vi "output.vi"(8 "error in (no error)":errorcluster, 10 "Output [on/off]":bool, 11 "PSP-603 in":refnum<class "PSP-603.lvclass">) -> (0 "error out":errorcluster, 3 "PSP-603 out":refnum<class "PSP-603.lvclass">)   [LabVIEW 2025, in "Power Supply.lvlib" / "PSP-603.lvclass"]
uses:
  PSP-603.lvclass
  PSP-603.lvclass/PSP-603.ctl
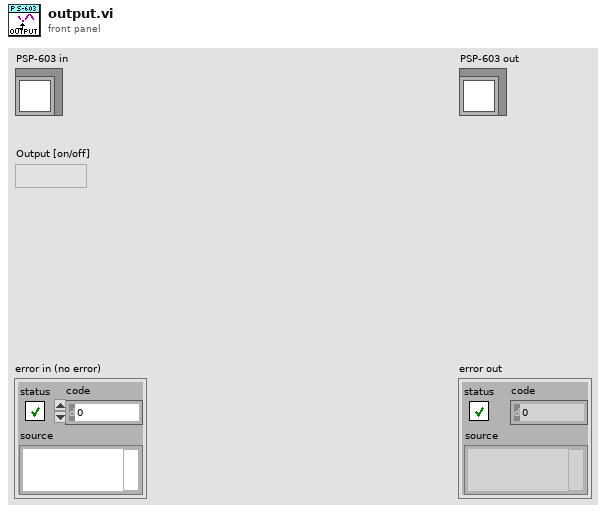
[diagram p1: front panel]
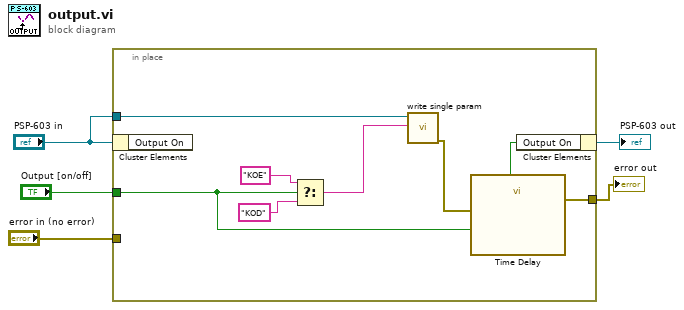
[diagram p0: block diagram]
diagram:
  n1 = in-place {
    in-place-border: "Output [on/off]" -> [w11]
    in-place-border: "PSP-603 in" -> [w12]
    in-place-border: "error in (no error)" -> [_]
    in-place-border: [w6] -> w1
    n2 = in-place-cluster #1("PSP-603 in") -> ()  [unwired: 1 out]
    n3 = Select(t="KOE" ("string"), s=w11, f="KOD" ("string")) -> (s? t:f=w8:string)
    n4 = call-dynamic "write single param.vi"("string"=w8, "PSP-603 in"=w12) -> ("error out"=w7:errorcluster)  [unwired: 8 in, 1 out]
    n5 = call "Time Delay"("error in (no error)"=w7) -> ("error out"=w6:errorcluster)  [unwired: 10 in]
    n6 = in-place-cluster #1("Output On"=w11) -> (→"PSP-603 out":refnum<class "PSP-603.lvclass">)
  }
  "error out" <- w1
